vi "Zen8OP500_refaire_P.vi"(1 "image":string, 5 "refaire":T1=enum."Scan", 6 "Pédale":bool, 7 "casOK":T1=enum."Crash", 8 "errin":errorcluster, 9 "test ok ?":bool, 10 "MSG Jerome":string, 11 "Visa Pedale":refnum<visa-resource-name>) -> (0 "errout":errorcluster, 3 "Next":T1=enum."Crash")   [LabVIEW 2020]
uses:
  OP500Z8_state_P.ctl
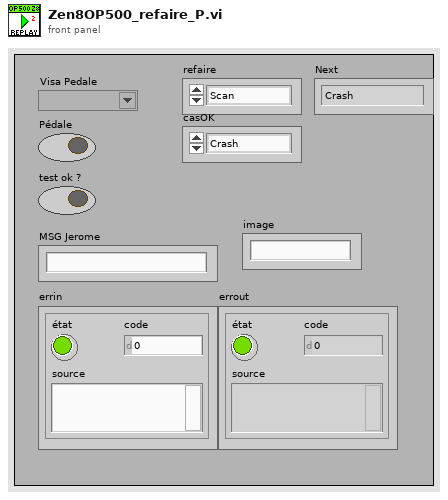
[diagram p1: front panel]
types:
  T1 = typedef "OP500Z8_state_P.ctl" = enum16{"Null", "Demarrage", "Init", "Scan", "Montage", "OCV", "Conti", "Iso", "CANCOM", "GoDCIR", "DataDyn", "Demontage", "Crash", "Next", "DCIR", "EXIT", "LogErr", "DTC"}
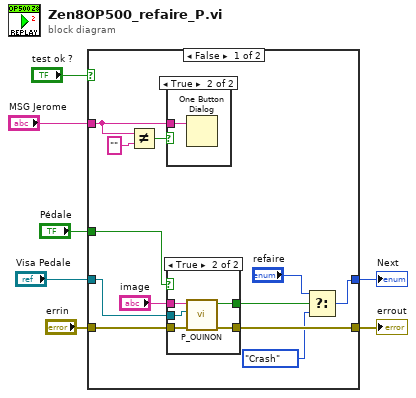
[diagram p0: block diagram]
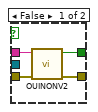
[diagram p3: hidden frame]
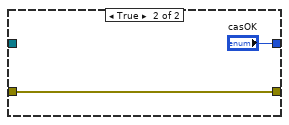
[diagram p4: hidden frame]
diagram:
  n1 = case shown="False" "test ok ?" {
    tunnel: "errin" -> [w19 w31]
    tunnel: [w18 w31] -> w7
    tunnel: "Visa Pedale" -> [w17 _]
    tunnel: "MSG Jerome" -> [w13 _]
    tunnel: "Pédale" -> [w16 _]
    tunnel: [w8 "casOK"] -> w1
    frame False {
      n2 = Not Equal?(x=w13, y="") -> (x != y?=w11:bool)
      n3 = case shown="True" w11 {
        tunnel: w13 -> [_ w20]
        frame False {
        }
        frame True {
          n4 = One Button Dialog(message=w20) -> ()  [unwired: 1 in, 1 out]
        }
      }
      n5 = case shown="True" w16 {
        tunnel: "image" -> [w21 w29]
        tunnel: w19 -> [w24 w28]
        tunnel: [w23 w27] -> w18
        tunnel: [w22 w26] -> w14
        tunnel: w17 -> [_ w25]
        frame False {
          n6 = call <userlib>:"OUINONV2.vi"("errin"=w24, "image"=w21) -> ("error out"=w23:errorcluster, "Booléen"=w22:bool)  [unwired: 8 in]
        }
        frame True {
          n7 = call "P_OUINON.vi"("errin"=w28, "VISAin"=w25, "Image"=w29) -> ("error out"=w27:errorcluster, "=OUI?"=w26:bool)  [unwired: 7 in]
        }
      }
      n8 = Select(t="refaire", s=w14, f=OP500Z8_state_P."Crash" ("Énum")) -> (s? t:f=w8:T1)
    }
    frame True {
    }
  }
  "errout" <- w7
  "Next" <- w1
